vi "SaveGroupAverages.vi"(8 "nAverages":u32=12, 9 "Value":u16, 11 "Complex":cluster{dbl, "df":dbl, cdb[]}[](array[cluster])) -> (2 "New Path":path)   [LabVIEW 2022 SP3]
uses:
  Mic/Mic_Global.vi
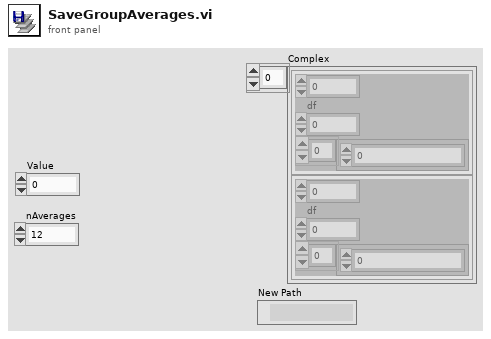
[diagram p1: front panel]
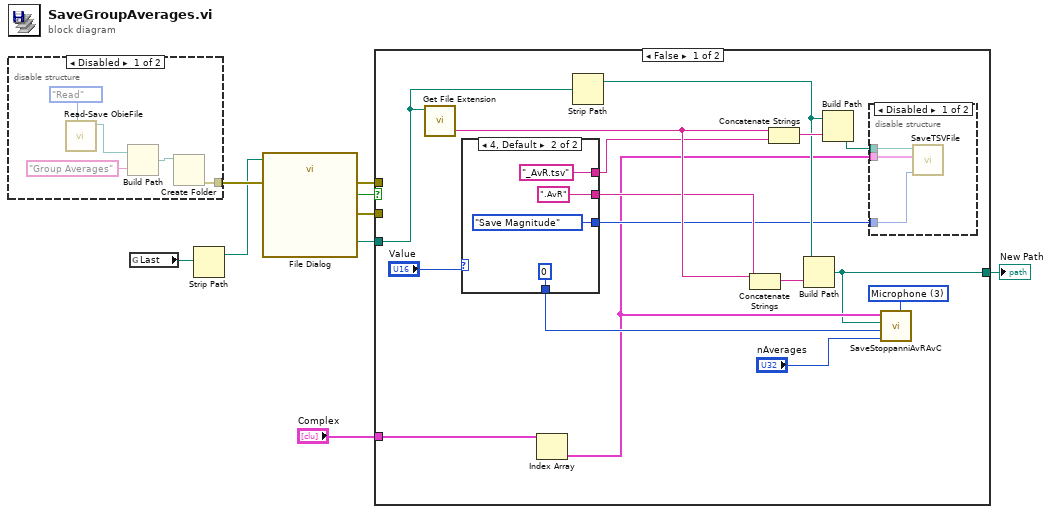
[diagram p0: block diagram]
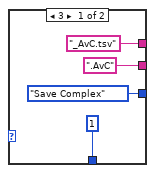
[diagram p4: hidden frame]
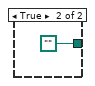
[diagram p5: hidden frame]
diagram:
  n1 = disable-structure shown="Disabled" {
    disable-tunnel: [w9 _] -> w5
    frame Disabled {
      n2 = call "Read-Save ObieFile.vi"("Task"=enum16{"Save", "Read"}."Read") -> ("DataPath Out"=w12:path)  [unwired: 8 in, 2 out]
      n3 = Build Path(base path=w12, name or relative path="Group Averages") -> (appended path=w10:path)
      n4 = Create Folder(path (use dialog)=w10) -> (error out=w9:errorcluster)  [unwired: 2 in, 2 out]
    }
    frame Enabled {
    }
  }
  n5 = global read "Mic_Global.vi" "Last"() -> (w2:path)
  n6 = Strip Path(path=w2) -> (stripped path=w1:path)  [unwired: 1 out]
  n7 = call "File Dialog"("start path"=w1) -> ("selected path"=w7:path, "cancelled"=w8:bool, "error out"=w6:errorcluster)  [unwired: 11 in, 1 out]
  n8 = case shown="False" w8 {
    tunnel: w7 -> [w25 _]
    tunnel: w6 -> [_ _]
    tunnel: w5 -> [_ _]
    tunnel: "Complex" -> [w16 _]
    tunnel: [w14 path ""] -> w3
    frame False {
      w19 = u8 3 items=["Accelerance", "Mobility", "Receptance", "Microphone", "Unknown"] ("dtAccel")
      n9 = call <vilib>:"Get File Extension.vi"("file"=w25) -> ("filename without extension"=w26:string)  [unwired: 6 in, 4 out]
      n10 = case shown="4, Default" "Value" {
        tunnel: ["_AvC.tsv" ("string") "_AvR.tsv" ("string")] -> w22
        tunnel: [".AvC" ("string") ".AvR" ("string")] -> w21
        tunnel: [1 0] -> w20
        tunnel: [enum16{"Save Magnitude", "Save Complex"}."Save Complex" ("Task") enum16{"Save Magnitude", "Save Complex"}."Save Magnitude" ("Task")] -> w17
        frame 3 {
        }
        frame 4, Default {
        }
      }
      n11 = Index Array(array=w16) -> (element=w15:cluster{dbl, "df":dbl, cdb[]})  [unwired: 1 in]
      n12 = Strip Path(path=w25) -> (stripped path=w24:path)  [unwired: 1 out]
      n13 = Concatenate Strings(w26, w21) -> (w27:string)
      n14 = Concatenate Strings(w26, w22) -> (w29:string)
      n15 = Build Path(base path=w24, name or relative path=w27) -> (appended path=w14:path)
      n16 = Build Path(base path=w24, name or relative path=w29) -> (appended path=w28:path)
      n17 = disable-structure shown="Disabled" {
        disable-tunnel: w28 -> [w32 _]
        disable-tunnel: w17 -> [w31 _]
        disable-tunnel: w15 -> [w30 _]
        frame Disabled {
          n18 = call "SaveTSVFile.vi"("Task"=w31, "FRF"=w30, "Path"=w32) -> ()  [unwired: 8 in, 1 out]
        }
        frame Enabled {
        }
      }
      n19 = call "SaveStoppanniAvRAvC.vi"("dtAccel"=w19, "nAverages"="nAverages", "fComplex"=w20, "file (use dialog)"=w14, "Complex FRF"=w15) -> ()  [unwired: 6 in, 1 out]
    }
    frame True {
    }
  }
  "New Path" <- w3
